vi "AI Acquire.vi"(8 "error in (no error)":errorcluster, 11 "Data Cluster in":T1 {"AI Config Data"."Analog Input Timing"."sample mode" items=["Finite Samples"=10178, "Continuous Samples"=10123, "Hardware Timed Single Point"=12522]}) -> (0 "error out":errorcluster, 2 "Stop":bool)   [LabVIEW 2024]
uses:
  Controls/Analog Input SM Data Cluster.ctl
  Analog Output/Controls/AIO Command Q Cluster.ctl
  Analog Output/Controls/AO Interface Data Cluster.ctl
  Analog Output/Controls/AO Channel Configuration Cluster.ctl
  Analog Output/Controls/AO Timing Cluster.ctl
  Main Engine/Controls/Main Engine JSON Command State.ctl
  TCP Engine/Controls/TCP Engine I&O  Interupt Cluster.ctl
  Host-DQMH/Configuration/Analog Input Single Channel Data--Cluster.ctl
  Host-DQMH/Configuration/Config-Channel Type.ctl
  Host-DQMH/Configuration/Channel Sub-Type.ctl
  Host-Control's/TCP Tx-Rx cluster.ctl
  <vilib>/DAQmx/read.llb/DAQmx Read (Analog 1D Wfm NChan NSamp).vi
  <vilib>/Analysis/baseanly.llb/Mean (DBL).vi
  <vilib>/DAQmx/read.llb/DAQmx Read (Analog 1D DBL NChan 1Samp).vi
  <vilib>/DAQmx/miscellaneous.llb/DAQmx Fill In Error Info.vi
  <vilib>/addons/_JKI.lib/Serialization/JSON/JKI JSON Serialization.lvlib
  <vilib>/Analysis/NI_AALBase.lvlib
  RT-DQMH-Module's/RT-TDMS-Logging/RT-TDMS-Logging.lvlib
  TCP Engine/TCP Engine.lvlib
  Host-DQMH/Configuration/Configuration.lvlib
panel:
  out "Actual Sampling Rate":dbl
  out "Timing.samples per channel":i32
  out "While Loop Duration(ms)":u32
  out "Daq mx Read Rate":dbl
  out "ms  to Wait":u32
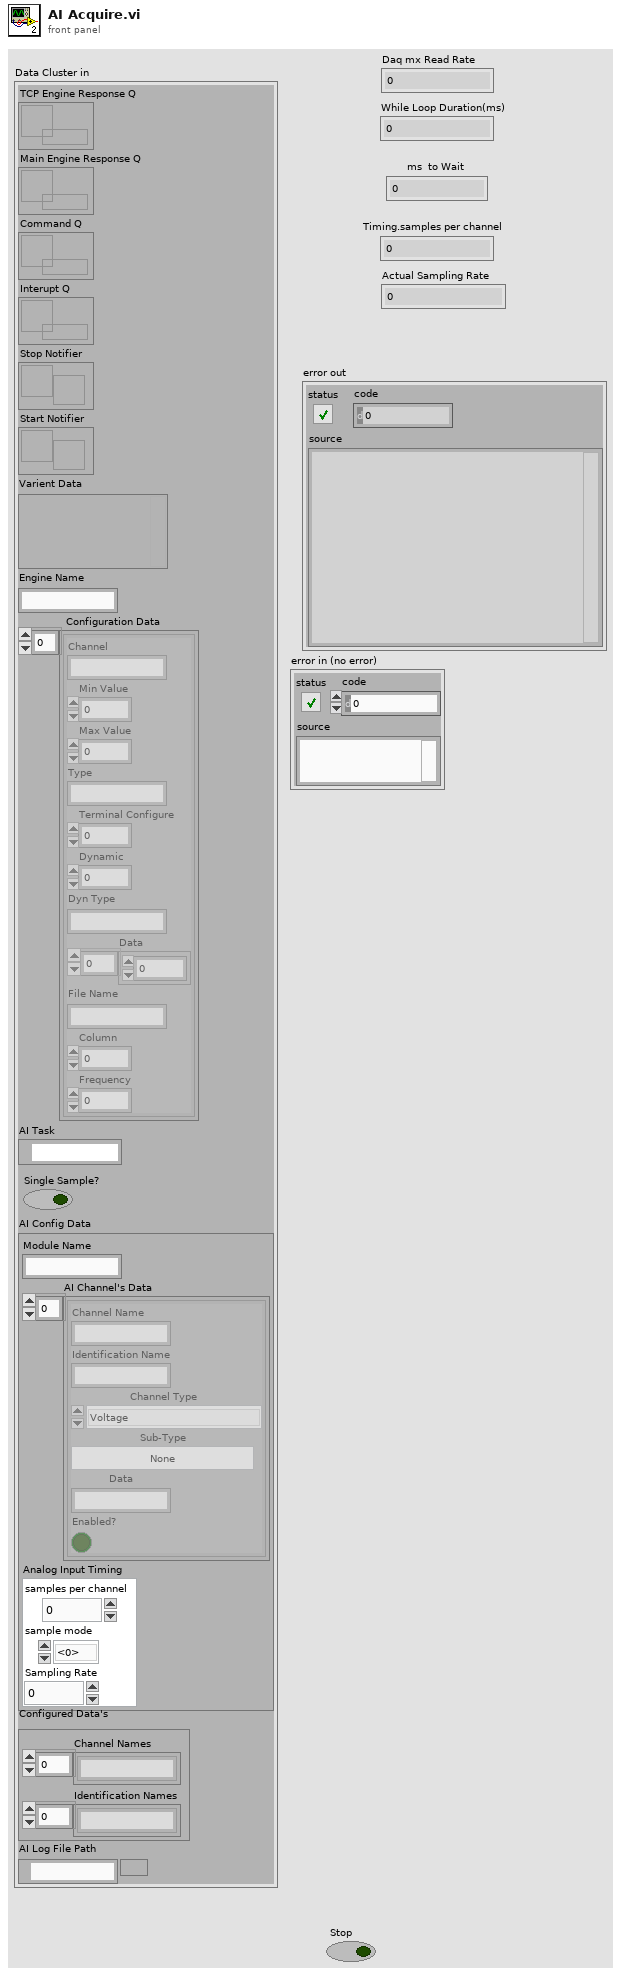
[diagram p1: front panel]
types:
  T1 = typedef "Analog Input SM Data Cluster.ctl" = cluster{"TCP Engine Response Q":refnum<queue>, "Main Engine Response Q":refnum<queue>, "Command Q":refnum<queue>, "Interupt Q":refnum<queue>, "Stop Notifier":refnum<notifier>, "Start Notifier":refnum<notifier>, "Varient Data":variant, "Engine Name":string, "Configuration Data":T2[], "AI Task":refnum<k21>, "Single Sample?":bool, "AI Config Data":cluster{"Module Name":string, "AI Channel's Data":T3[], "Analog Input Timing":T6}, "Configured Data's":cluster{"Channel Names":string[], "Identification Names":string[]}, "AI Log File Path":path}
  T2 = typedef "AO Channel Configuration Cluster.ctl" = cluster{"Channel":string, "Min Value":dbl, "Max Value":dbl, "Type":string, "Terminal Configure":u16, "Dynamic":u8, "Dyn Type":string, "Data":dbl[], "File Name":string, "Column":i32, "Frequency":dbl}
  T3 = typedef "Configuration.lvlib/Analog Input Single Channel Data--Cluster.ctl" = cluster{"Channel Name":string, "Identification Name":string, "Channel Type":T4, "Sub-Type":T5, "Data":string, "Enabled?":bool}
  T4 = typedef "Configuration.lvlib/Config-Channel Type.ctl" = enum16{"Voltage", "Current", "Thermocouple", "Acclerometer"}
  T5 = typedef "Configuration.lvlib/Channel Sub-Type.ctl" = enum16{"None", "Pressure", "Force"}
  T6 = typedef "AO Timing Cluster.ctl" = cluster{"samples per channel":i32, "sample mode":i32, "Sampling Rate":dbl}
  T7 = typedef "TCP Tx-Rx cluster.ctl" = cluster{"Interface":string, "Command":string, "SubCmd":string, "Data":variant}
  T8 = cluster{"Channel":string, "Data":dbl, "Data & Time":string}
  T9 = cluster{"String":string, "Waveform":waveform(dbl), "date/time string":string}[]
  T10 = cluster{"Channel":string, "Data":waveform(dbl), "Time":timestamp}[]
  T11 = cluster{timestamp[], "Identification Names":string[], dbl[]}
  T12 = cluster{"String":string, "mean":dbl, "date/time string":string}[]
  T13 = cluster{"String":string, "Waveform":dbl, "date/time string":string}[]
  T14 = cluster{"Channel":string, "Data":dbl, "Time":timestamp}[]
  T15 = cluster{"Identification Names":string[], "data":dbl[]}
  T16 = typedef "TCP Engine.lvlib/TCP Engine I&O  Interupt Cluster.ctl" = cluster{" Stop":bool, "JSON Variant":variant}
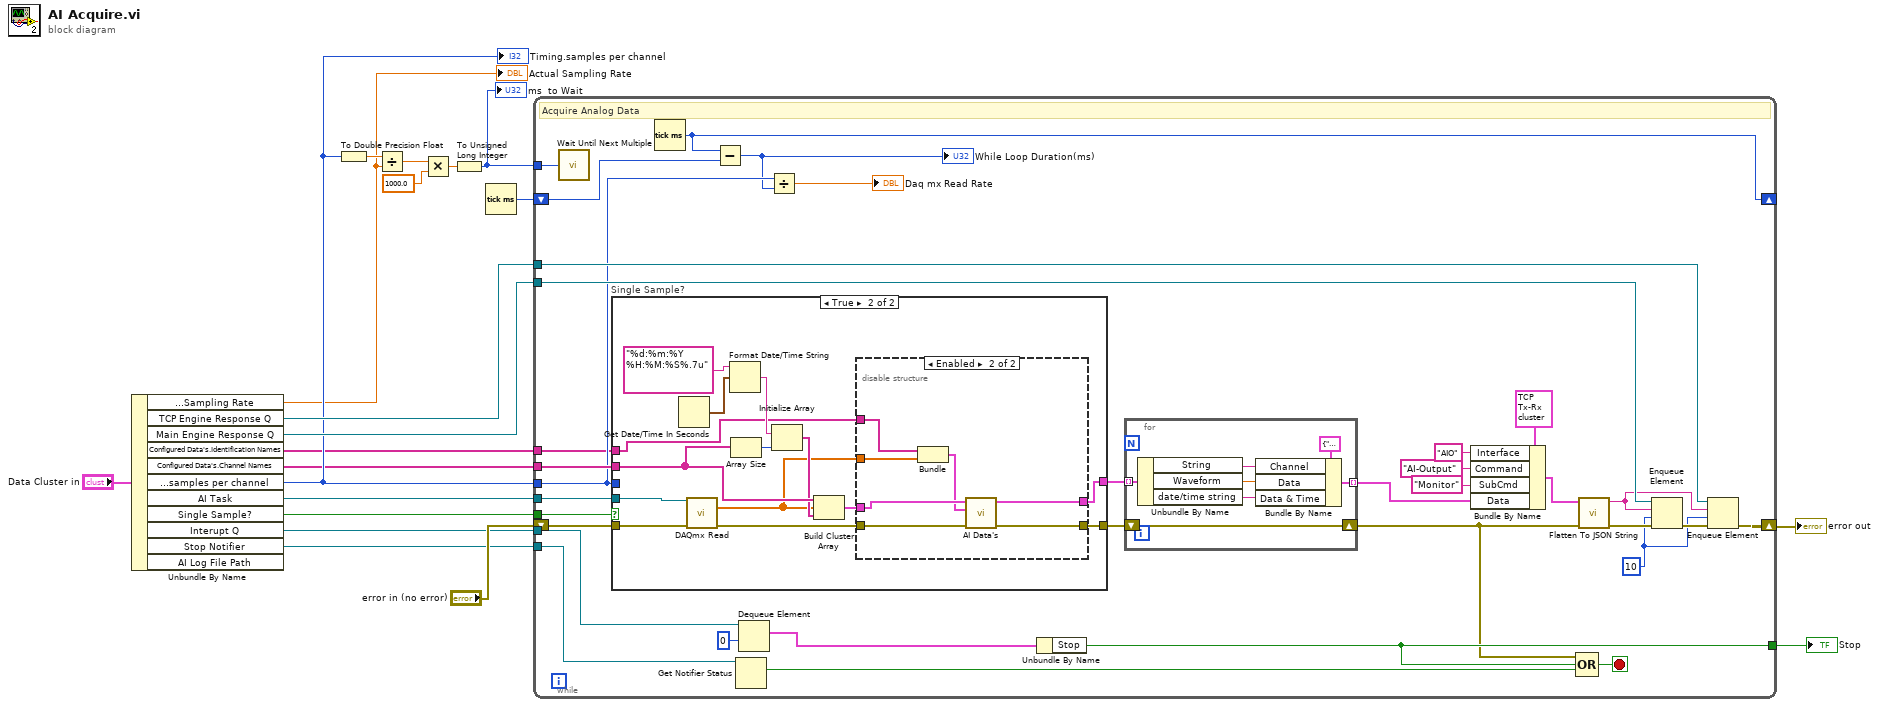
[diagram p0: block diagram]
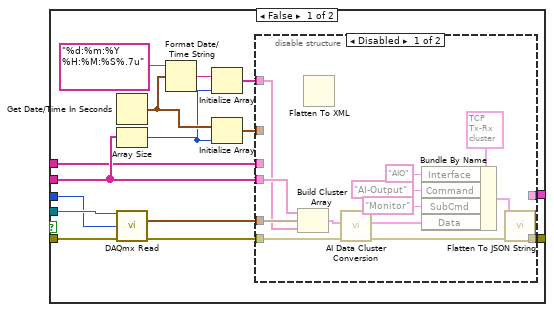
[diagram p2: hidden frame]
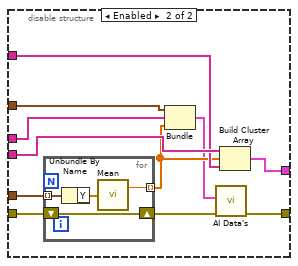
[diagram p3: hidden frame]
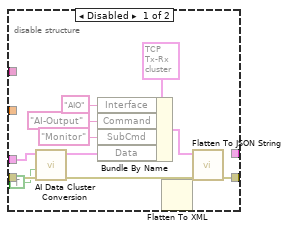
[diagram p4: hidden frame]
diagram:
  n1 = Unbundle By Name("Data Cluster in") -> ("AI Config Data.Analog Input Timing.Sampling Rate"=w3:dbl, "TCP Engine Response Q"=w10:refnum<queue>, "Main Engine Response Q"=w11:refnum<queue>, "Configured Data's.Identification Names"=w1:string[], "Configured Data's.Channel Names"=w2:string[], "AI Config Data.Analog Input Timing.samples per channel"=w6:i32, "AI Task"=w12:refnum<k21>, "Single Sample?"=w13:bool, "Interupt Q"=w14:refnum<queue>, "Stop Notifier"=w15:refnum<notifier>)  [unwired: 1 out]
  "Timing.samples per channel" <- w6
  "Actual Sampling Rate" <- w3
  n2 = To Double Precision Float(number=w6) -> (double precision float=w4:dbl)
  n3 = Divide(x=w4, y=w3) -> (x/y=w19:dbl)
  n4 = Multiply(x=w19, y=1000.0) -> (x*y=w8:dbl)
  n5 = To Unsigned Long Integer(number=w8) -> (unsigned 32bit integer=w5:u32)
  "ms  to Wait" <- w5
  n6 = Tick Count (ms)() -> (millisecond timer value=w7:u32)
  n7 = while {
    tunnel: w10 -> [w48]
    tunnel: w11 -> [w49]
    tunnel: w12 -> [w53]
    tunnel: w13 -> [w54]
    tunnel: w14 -> [w52]
    tunnel: w15 -> [w24]
    tunnel: w6 -> [w39]
    tunnel: [w45] -> w17
    tunnel: w2 -> [w42]
    shift-right: [w41] -> _
    shift-left: w7 -> [w40]
    tunnel: w5 -> [w36]
    shift-right: [w46] -> w16
    shift-left: "error in (no error)" -> [w44]
    tunnel: w1 -> [w22]
    stop <- w51 stop-if-true
    w21 = 10 ("timeout in ms (-1)")
    # "Acquire Analog Data"
    n8 = call "Wait Until Next Multiple"("Count(mSec)"=w36) -> ()  [unwired: 1 out]
    n9 = case "Single Sample?" shown="True" w54 {
      tunnel: w53 -> [w75 w118]
      tunnel: w44 -> [w76 w117]
      tunnel: [w73 w116] -> w31
      tunnel: w39 -> [w74 _]
      tunnel: w42 -> [w70 w114]
      tunnel: [w68 w110] -> w30
      tunnel: w22 -> [w65 w106]
      frame False {
        n10 = Get Date/Time In Seconds() -> (seconds since 1Jan1904=w64:timestamp)
        n11 = Array Size(array=w70) -> (size(s)=w63:i32)
        n12 = call-poly <vilib>:"DAQmx Read.vi"("task/channels in"=w75, "number of samples per channel"=w74, "error in"=w76) -> ("data"=w72:waveform(dbl)[], "error out"=w71:errorcluster)  [unwired: 10 in, 1 out]
        n13 = Format Date/Time String(time format string (%c)="%d:%m:%Y %H:%M:%S%.7u", seconds (now)=w64) -> (date/time string=w66:string)  [unwired: 1 in]
        n14 = Initialize Array(w66, w63) -> (w69:string[])
        n15 = Initialize Array(w64, w63) -> (w62:timestamp[])
        n16 = disable-structure shown="Disabled" {
          disable-tunnel: [w89 w94] -> w73
          disable-tunnel: w72 -> [w88 w100]
          disable-tunnel: w71 -> [w87 w99]
          disable-tunnel: w70 -> [w85 w98]
          disable-tunnel: w69 -> [w77 w97]
          disable-tunnel: [_ w96] -> w68
          disable-tunnel: w65 -> [_ w93]
          disable-tunnel: w62 -> [_ w91]
          frame Disabled {
            n17 = Build Cluster Array ("Index & Bundle Cluster Array")(w85, w88, w77) -> (w78:T9)
            n18 = Flatten To XML() -> ()  [unwired: 1 in, 1 out]
            n19 = call "AI Data Cluster Conversion.vi"("error in"=w87, "Waveform Cluster"=w78) -> ("error out"=w86:errorcluster, "Waveform Array"=w79:T10)  [unwired: 7 in, 1 out]
            n20 = Bundle By Name(cluster=T7 {"Interface"="CPU", "Command"="CPU Info", "SubCmd"="Monitor", "Data"=variant} ("TCP Tx-Rx Cluster"), "Interface"="AIO", "Command"="AI-Output", "SubCmd"="Monitor" ("Sub Cmd"), "Data"=w79) -> (w80:T7)
            n21 = call <vilib>:"Flatten To JSON String.vi"("error in"=w86, "Variant"=w80) -> ("error out"=w89:errorcluster)  [unwired: 8 in, 1 out]
          }
          frame Enabled {
            n22 = for {
              tunnel: w100 -> [w104] mode=indexing
              tunnel: [w101] -> w92 mode=indexing
              shift-right: [w103] -> w95
              shift-left: w99 -> [w103]
              n23 = Unbundle By Name(w104) -> ("Y"=w102:dbl[])
              n24 = call-poly <vilib>:"Mean.vi"("X"=w102) -> ("mean"=w101:dbl)  [unwired: 1 out]
            }
            n25 = Bundle(w91, "Identification Names"=w93, w92) -> (w90:T11)  [unwired: 1 in]
            n26 = call "AI Data's.vi"("error in"=w95, "AI Data's"=w90) -> ("error out"=w94:errorcluster)  [unwired: 9 in]
            n27 = Build Cluster Array ("Index & Bundle Cluster Array")(w98, w92, w97) -> (w96:T12)
          }
        }
      }
      frame True {
        n28 = Get Date/Time In Seconds() -> (seconds since 1Jan1904=w108:timestamp)
        n29 = call-poly <vilib>:"DAQmx Read.vi"("task/channels in"=w118, "error in"=w117) -> ("data"=w105:dbl[], "error out"=w115:errorcluster)  [unwired: 11 in, 1 out]
        n30 = Format Date/Time String(time format string (%c)="%d:%m:%Y %H:%M:%S%.7u", seconds (now)=w108) -> (date/time string=w107:string)  [unwired: 1 in]
        n31 = Array Size(array=w114) -> (size(s)=w113:i32)
        n32 = Initialize Array(w107, w113) -> (w112:string[])
        n33 = Build Cluster Array ("Index & Bundle Cluster Array")(w114, w105, w112) -> (w111:T13)
        n34 = disable-structure shown="Enabled" {
          disable-tunnel: [w129 w131] -> w116
          disable-tunnel: w115 -> [w128 w132]
          disable-tunnel: w111 -> [w126 w135]
          disable-tunnel: [_ w135] -> w110
          disable-tunnel: w106 -> [_ w134]
          disable-tunnel: w105 -> [_ w133]
          frame Disabled {
            n35 = call "AI Data Cluster Conversion.vi"("error in"=w128, "1D array?"=TRUE, "Input 1D Cluster"=w126) -> ("error out"=w125:errorcluster, "1D Array"=w119:T14)  [unwired: 6 in, 1 out]
            n36 = Bundle By Name(cluster=T7 {"Interface"="CPU", "Command"="CPU Info", "SubCmd"="Monitor", "Data"=variant} ("TCP Tx-Rx Cluster"), "Interface"="AIO", "Command"="AI-Output", "SubCmd"="Monitor" ("Sub Cmd"), "Data"=w119) -> (w120:T7)
            n37 = Flatten To XML() -> ()  [unwired: 1 in, 1 out]
            n38 = call <vilib>:"Flatten To JSON String.vi"("error in"=w125, "Variant"=w120) -> ("error out"=w129:errorcluster)  [unwired: 8 in, 1 out]
          }
          frame Enabled {
            n39 = Bundle("Identification Names"=w134, "data"=w133) -> (w130:T15)  [unwired: 1 in]
            n40 = call "AI Data's.vi"("error in"=w132, "AI Data's"=w130) -> ("error out"=w131:errorcluster)  [unwired: 9 in]
          }
        }
      }
    }
    n41 = Tick Count (ms)() -> (millisecond timer value=w41:u32)
    n42 = Subtract(x=w41, y=w40) -> (x-y=w37:u32)
    "While Loop Duration(ms)" <- w37
    n43 = Get Notifier Status(notifier=w24) -> (current notification=w23:bool)  [unwired: 1 in, 4 out]
    n44 = Dequeue Element(queue=w52, timeout in ms (-1)=0) -> (element=w50:T16)  [unwired: 1 in, 3 out]
    n45 = Divide(x=w39, y=w37) -> (x/y=→"Daq mx Read Rate":dbl)
    n46 = Unbundle By Name(w50) -> ("Stop"=w45:bool)
    n47 = for {
      tunnel: w30 -> [w61] mode=indexing
      shift-right: [w56] -> w27
      shift-left: w31 -> [w56]
      tunnel: [w55] -> w29 mode=indexing
      n48 = Unbundle By Name(w61) -> ("String"=w60:string, "Waveform"=w59:dbl, "date/time string"=w58:string)
      n49 = Bundle By Name(cluster=T8 {"Channel"="", "Data"=0.0, "Data & Time"=""} ("Cluster"), "Channel"=w60, "Data"=w59, "Data & Time"=w58) -> (w55:T8)
    }
    n50 = Bundle By Name(cluster=T7 {"Interface"="CPU", "Command"="CPU Info", "SubCmd"="Monitor", "Data"=variant} ("TCP Tx-Rx Cluster"), "Interface"="AIO", "Command"="AI-Output", "SubCmd"="Monitor" ("Sub Cmd"), "Data"=w29) -> (w28:T7)
    n51 = Compound Arithmetic op=OR(w27, w45, w23) -> (w51:bool)
    n52 = call <vilib>:"Flatten To JSON String.vi"("error in"=w27, "Variant"=w28) -> ("error out"=w26:errorcluster, "JSON String"=w25:string)  [unwired: 8 in]
    n53 = Enqueue Element(queue=w49, element=w25, timeout in ms (-1)=w21, error in (no error)=w26) -> (error out=w47:errorcluster)  [unwired: 2 out]
    n54 = Enqueue Element(queue=w48, element=w25, timeout in ms (-1)=w21, error in (no error)=w47) -> (error out=w46:errorcluster)  [unwired: 2 out]
  }
  "Stop" <- w17
  "error out" <- w16
